vi "EAGLE GUI V2.vi"() -> ()   [LabVIEW 2015]
panel:
  in  "Play Button":bool
  in  "String 2":string
  out "Image":T1(plugin-control)
  in  "String":string
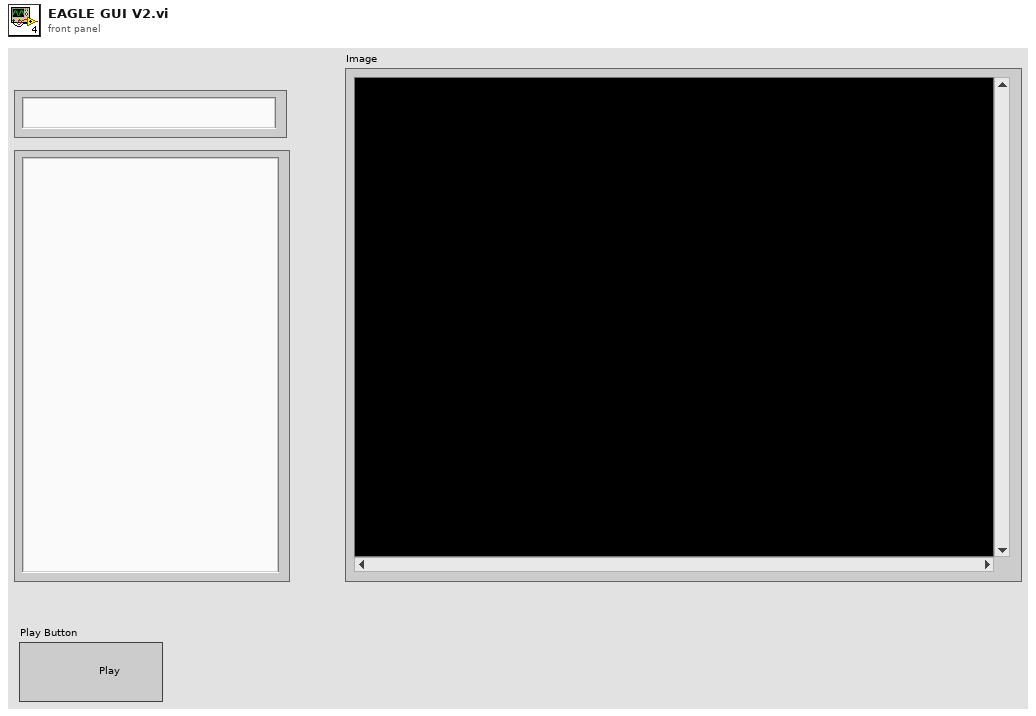
[diagram p1: front panel]
types:
  T1 = typedef "IMAQ Image.ctl" = refnum<image>
  T2 = typedef "LVRectTypeDef.ctl" = cluster{"Left":i16, "Top":i16, "Right":i16, "Bottom":i16}
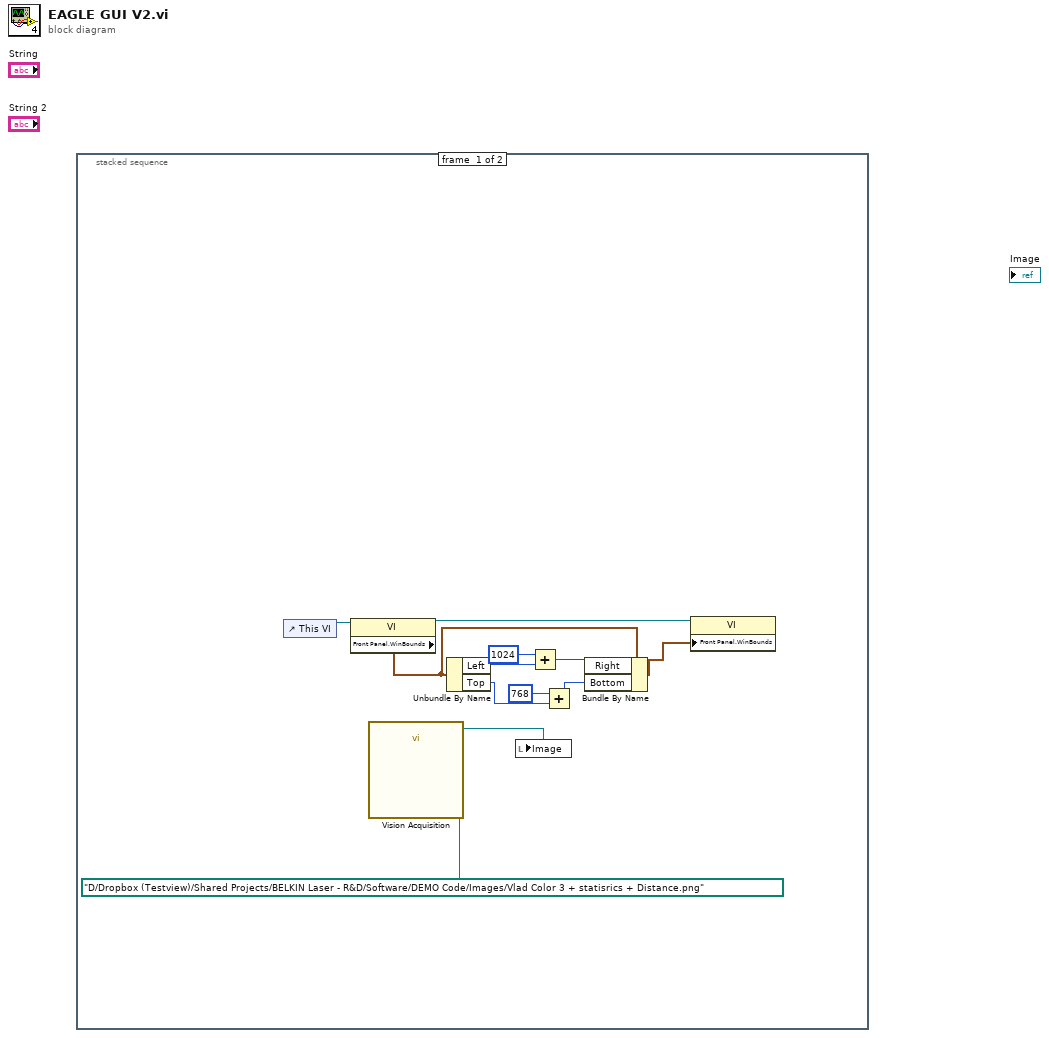
[diagram p0: block diagram]
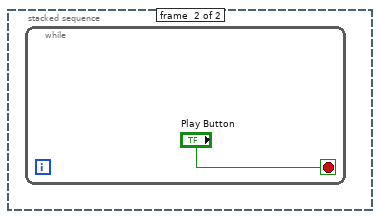
[diagram p2: hidden frame]
diagram:
  n1 = stacked-sequence {
    frame #0 {
      n2 = control-ref of="This VI"() -> (w11:refnum<vi>)
      n3 = property class="VI"(reference=w11) -> (reference out=w10:refnum<vi>, "Front Panel.WinBounds"=w9:T2)  [unwired: 1 in, 1 out]
      n4 = call "Vision Acquisition"("Image Path"=path "D:/Dropbox (Testview)/Shared Projects/BELKIN Laser - R&D/Software/DEMO Code/Images/Vlad Color 3 + statisrics + Distance.png") -> ("Image Out"=w1:T1)  [unwired: 25 in, 1 out]
      n5 = Unbundle By Name(w9) -> ("Left"=w8:i16, "Top"=w3:i16)
      n6 = local write "Image"(w1) -> ()
      n7 = Add(x=i16 1024, y=w8) -> (x+y=w6:i16)
      n8 = Add(x=i16 768, y=w3) -> (x+y=w4:i16)
      n9 = Bundle By Name(cluster=w9, "Right"=w6, "Bottom"=w4) -> (w2:T2)
      n10 = property class="VI"(reference=w10, "Front Panel.WinBounds"=w2) -> ()  [unwired: 1 in, 2 out]
    }
    frame #1 {
      n11 = while {
        stop <- "Play Button" stop-if-true
      }
    }
  }
